vi "Get Created.vi"(10 "Addresses DVR":refnum<data-value>) -> (0 "error out":errorcluster, 2 "Created":T1)   [LabVIEW 2021, in "jettl.lvlib" / "Addresses.lvlib"]
uses:
  Addresses.lvlib
  Addresses/Addresses.lvclass
  Msg Type Strategy/Msg Type Strategy/Msg Type Strategy.lvclass
  Created.ctl
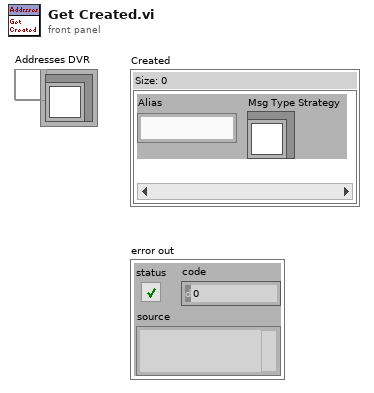
[diagram p1: front panel]
types:
  T1 = typedef "jettl.lvlib/Addresses.lvlib/Created.ctl" = map{string, refnum<class "Msg Type Strategy.lvclass">}
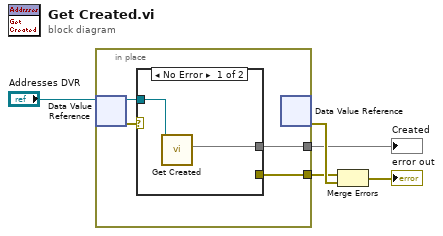
[diagram p0: block diagram]
diagram:
  n1 = in-place {
    in-place-border: [w9] -> w2
    in-place-border: [w8] -> w1
    n2 = in-place-dvr #1("Addresses DVR") -> (w6:refnum<class "Addresses.lvclass">, w7:errorcluster)
    n3 = case shown="No Error" w7 {
      selector: w7 -> [_ w12]
      tunnel: w6 -> [w11 _]
      tunnel: [_ w12] -> w9
      tunnel: [w10 _] -> w8
      frame No Error {
        n4 = call "Get Created.vi"("Addresses in"=w11) -> ("Created"=w10:T1)  [unwired: 10 in]
      }
      frame Error {
      }
    }
    n5 = in-place-dvr #1() -> (w3:errorcluster)  [unwired: 1 in, 1 out]
  }
  "Created" <- w1
  n6 = Merge Errors(w2, w3) -> (→"error out":errorcluster)
